vi "Final.vi"() -> ()   [LabVIEW 2017]
doc: "This example demonstrates how to read the hand position and velocity using the Leap Motion Controller."
uses:
  <vilib>/MakerHub/Leap/Private/Type Defs/Frame.ctl
  <vilib>/MakerHub/Leap/Private/Type Defs/Gesture Key Tap.ctl
  <vilib>/MakerHub/Leap/Private/Type Defs/Gesture Common.ctl
  <vilib>/MakerHub/Leap/Private/Type Defs/Gesture Type.ctl
  <vilib>/MakerHub/Leap/Private/Type Defs/Gesture State.ctl
  <vilib>/MakerHub/Leap/Private/Type Defs/Vector.ctl
  <vilib>/MakerHub/Leap/Private/Type Defs/Gesture Circle.ctl
  <vilib>/MakerHub/Leap/Private/Type Defs/Gesture Screen Tap.ctl
  <vilib>/MakerHub/Leap/Private/Type Defs/Gesture Swipe.ctl
  <vilib>/MakerHub/Leap/Private/Type Defs/Hand.ctl
  <vilib>/MakerHub/Leap/Private/Type Defs/Pointable.ctl
  <vilib>/MakerHub/Leap/Private/Type Defs/Pointable Type.ctl
  <vilib>/MakerHub/Leap/Private/Type Defs/Pointable Zone.ctl
  <vilib>/Instr/_visa.llb/VISA Configure Serial Port (Instr).vi
  <vilib>/MakerHub/Leap/Public/Instance VIs/Read 1 Hand Position Velocity.vi
  <vilib>/MakerHub/Leap/LMH-Leap.lvlib
panel:
  out "Hand XZ Position":cluster{"X":sgl, "Z":sgl, "Y":sgl}[](graph)
  out "Y Velocity (m/s) 2":sgl(slide) scale=2.0..-2.0
  out "X Velocity (m/s)":sgl(slide) scale=-2.0..2.0
  out "Z Velocity (m/s)":sgl(slide) scale=2.0..-2.0
  out "Hand XYZ Position":cluster{"X":sgl, "Y":sgl, "Z":sgl}
  out "error out":errorcluster
  out "error?":bool
  out "STRING_SEND_FINAL":string
  in  "COM Port":refnum<visa-resource-name>
  in  "baud rate (9600)":u32=9600
  in  "string":string
  out "Frame":T1
  out "Leap Connected?":bool
  in  "Stop Button":bool
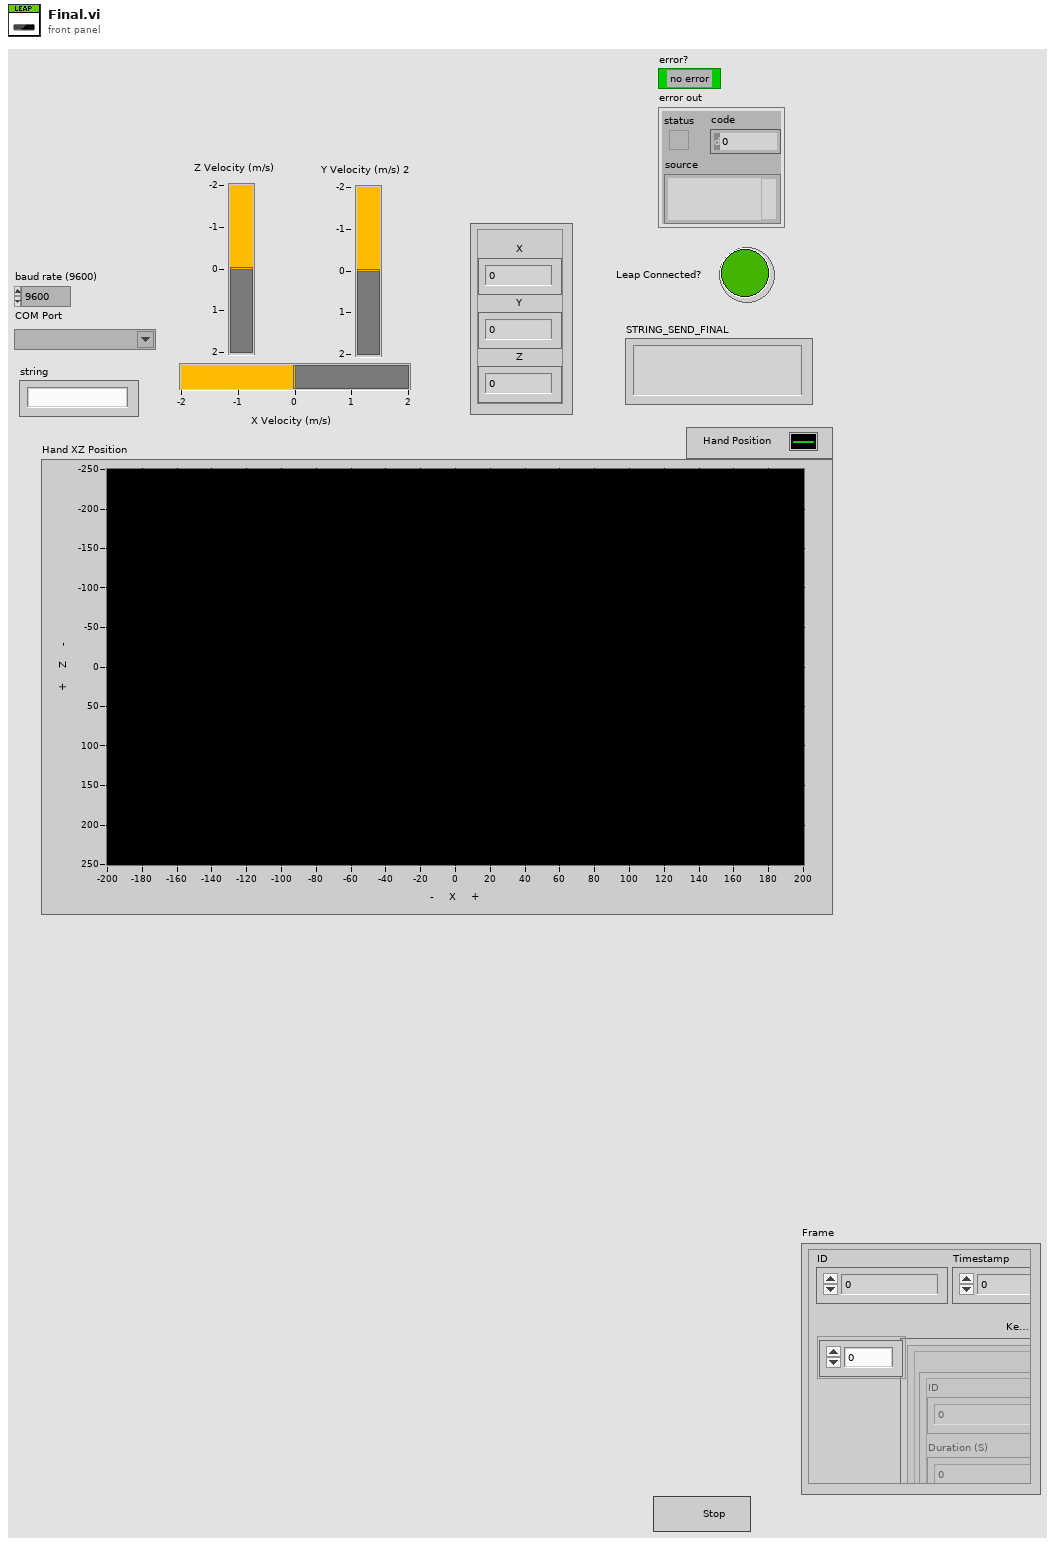
[diagram p1: front panel]
types:
  T1 = typedef "LMH-Leap.lvlib/Frame.ctl" = cluster{"ID":i64, "Timestamp":i64, "Current FPS":dbl, "Key Tap Gestures":T2[], "Circle Gestures":T7[], "Screen Tap Gestures":T8[], "Swipe Gestures":T9[], "Hands":T10[]}
  T2 = typedef "LMH-Leap.lvlib/Gesture Key Tap.ctl" = cluster{"Common":T3, "Direction":T6, "Position":T6, "Progress":dbl}
  T3 = typedef "LMH-Leap.lvlib/Gesture Common.ctl" = cluster{"ID":dbl, "Duration (S)":dbl, "Gesture Type":T4, "Gesture State":T5}
  T4 = typedef "LMH-Leap.lvlib/Gesture Type.ctl" = enum16{"Invalid", "Swipe", "Circle", "Screen Tap", "Key Tap"}
  T5 = typedef "LMH-Leap.lvlib/Gesture State.ctl" = enum16{"Invalid", "Start", "Update", "Stop"}
  T6 = typedef "LMH-Leap.lvlib/Vector.ctl" = cluster{"Pitch":sgl, "Yaw":sgl, "Roll":sgl, "Magnitude":sgl, "XYZ":sgl[]}
  T7 = typedef "LMH-Leap.lvlib/Gesture Circle.ctl" = cluster{"Common":T3, "Center":T6, "Normal":T6, "Progress":dbl, "Radius":dbl}
  T8 = typedef "LMH-Leap.lvlib/Gesture Screen Tap.ctl" = cluster{"Common":T3, "Direction":T6, "Position":T6, "Progress":dbl}
  T9 = typedef "LMH-Leap.lvlib/Gesture Swipe.ctl" = cluster{"Common":T3, "Direction":T6, "Position":T6, "Start Position":T6, "Speed":dbl}
  T10 = typedef "LMH-Leap.lvlib/Hand.ctl" = cluster{"Palm Normal":T6, "Palm Position":T6, "Palm Velocity":T6, "Direction":T6, "Palm Position (Stabilized)":T6, "Sphere Center":T6, "Pointables":T11[], "ID":i32, "Time Visible":sgl, "Sphere Radius":sgl}
  T11 = typedef "LMH-Leap.lvlib/Pointable.ctl" = cluster{"Type":T12, "Touch Zone":T13, "ID":i32, "Length":dbl, "Width":dbl, "Time Visible":dbl, "Touch Distance":dbl, "Direction":T6, "Tip Position":T6, "Tip Velocity":T6, "Tip Position (Stabilized)":T6}
  T12 = typedef "LMH-Leap.lvlib/Pointable Type.ctl" = enum16{"Finger", "Tool"}
  T13 = typedef "LMH-Leap.lvlib/Pointable Zone.ctl" = enum16{"None", "Hovering", "Touching"}
  T14 = typedef "LMH-Leap.lvlib/Leap Handle.ctl" = cluster{"LeapCSharp":refnum<k24>}
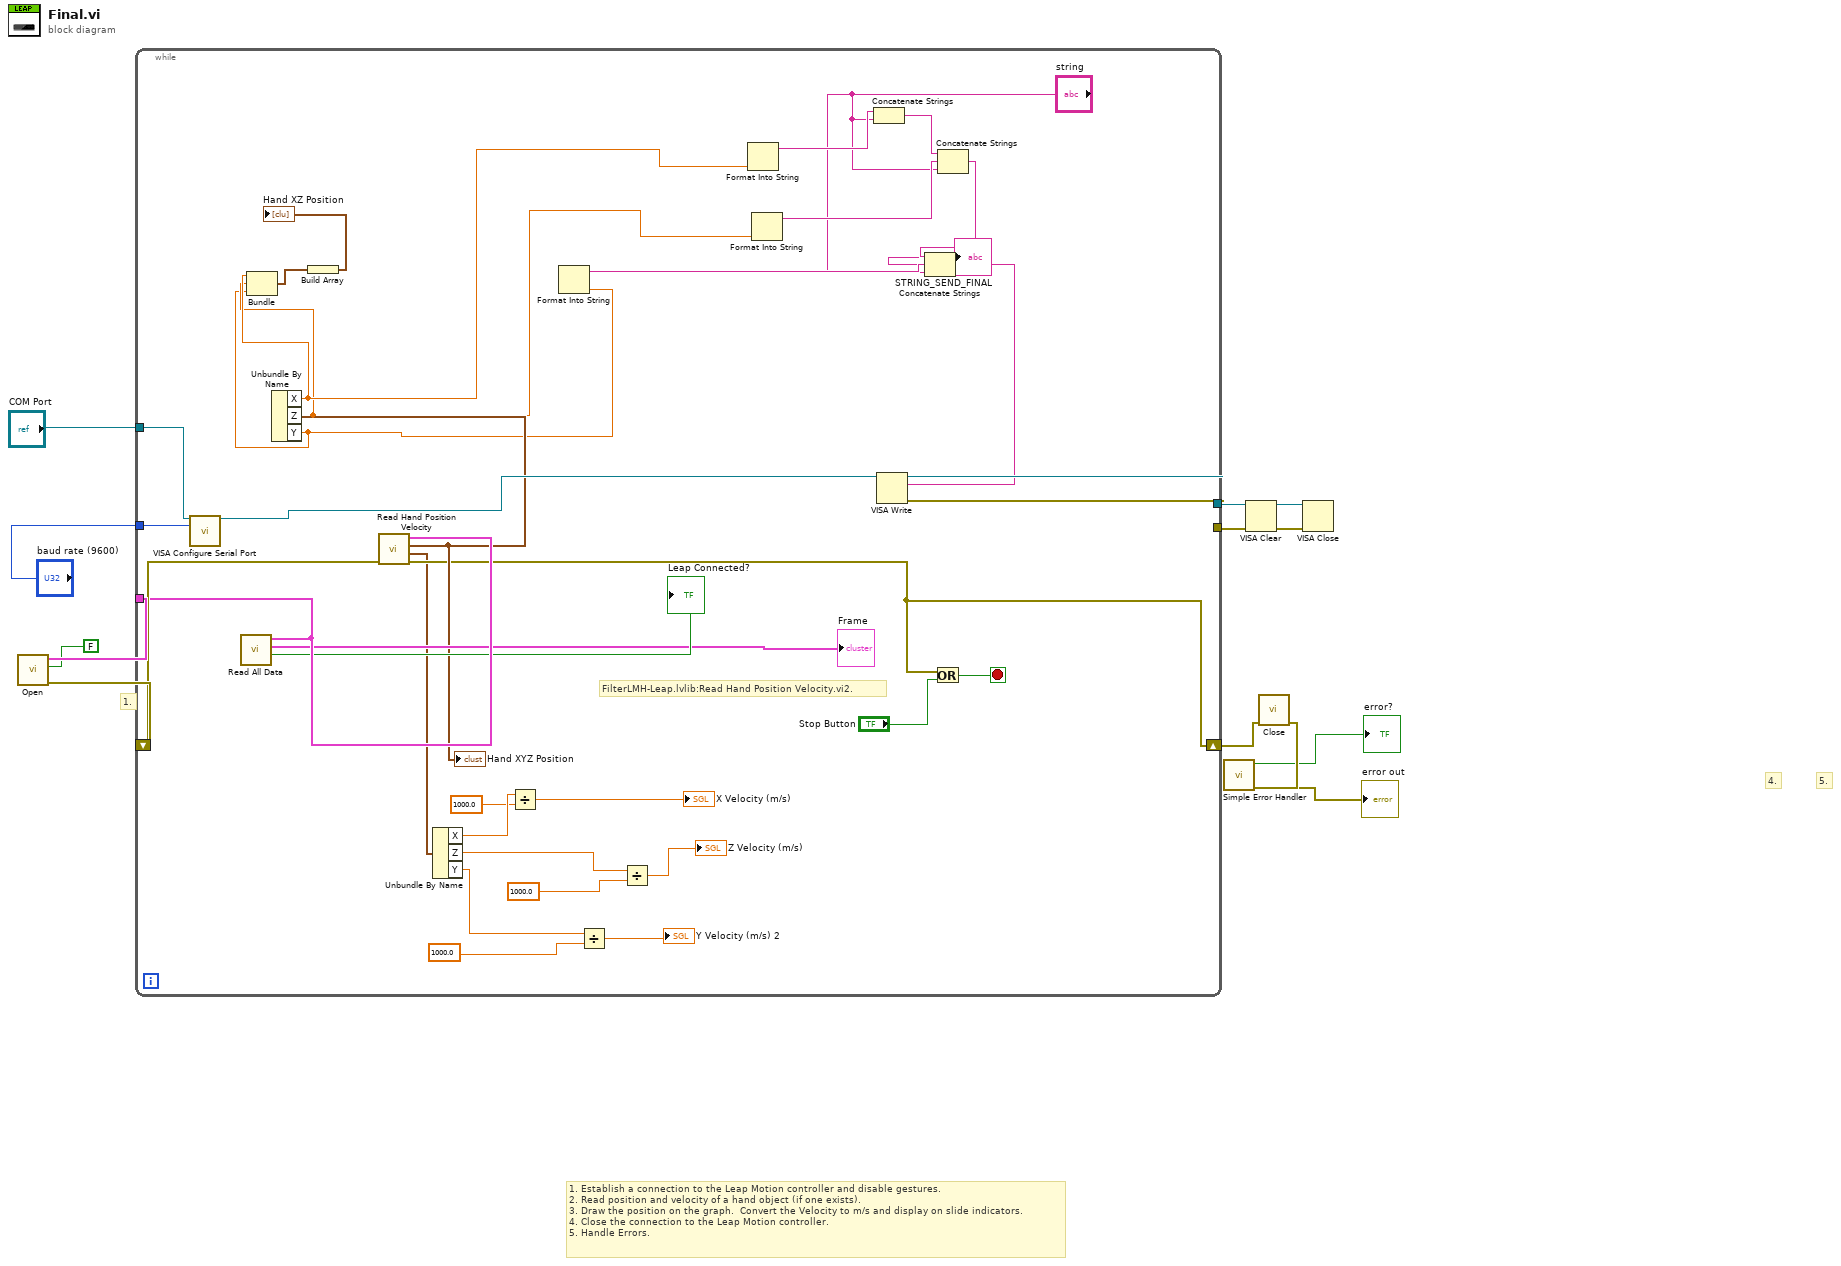
[diagram p0: block diagram]
diagram:
  # "1. Establish a connection to the Leap Motion controller and disable gestures.\n2. Read position and velocity of a hand object (if one exists).\n3. Draw the position on the graph.  Convert the Velocity to m/s and display on slide indicators.\n4. Close the connection to the Leap Motion controller.\n5. Handle Errors."
  # "5."
  # "4."
  # "1."
  n1 = call <vilib>:"Open.vi"("Enable Gestures? (T)"=FALSE) -> ("Error Out"=w12:errorcluster, "Leap Handle"=w13:T14)  [unwired: 9 in]
  n2 = while {
    tunnel: w13 -> [w45]
    shift-right: [w29] -> w4
    shift-left: w12 -> [w46]
    tunnel: [w42] -> w8
    tunnel: [w41] -> w6
    tunnel: "COM Port" -> [w40]
    tunnel: "baud rate (9600)" -> [w39]
    stop <- w48 stop-if-true
    # "FilterLMH-Leap.lvlib:Read Hand Position Velocity.vi2."
    n3 = call-poly "VISA Configure Serial Port"("VISA resource name"=w40, "baud rate (9600)"=w39) -> ("VISA resource name out"=w38:refnum<visa-resource-name>)  [unwired: 12 in, 1 out]
    n4 = call <vilib>:"Read All Data.vi"("Leap Handle"=w45) -> ("Leap Connected?"=→"Leap Connected?":bool, "Frame"=→"Frame":T1)  [unwired: 7 in, 2 out]
    n5 = call-poly <vilib>:"Read Hand Position Velocity.vi"("Error In"=w46, "Leap Handle"=w45) -> ("Error Out"=w29:errorcluster, "Hand Velocity"=w22:cluster{"X":sgl, "Y":sgl, "Z":sgl}, "Hand Position"=w30:cluster{"X":sgl, "Y":sgl, "Z":sgl})  [unwired: 6 in, 1 out]
    "Hand XYZ Position" <- w30
    n6 = Unbundle By Name(w30) -> ("X"=w18:sgl, "Z"=w17:sgl, "Y"=w16:sgl)
    n7 = Bundle("X"=w18, "Z"=w17, "Y"=w16) -> (w15:cluster{"X":sgl, "Z":sgl, "Y":sgl})  [unwired: 1 in]
    n8 = Build Array(w15) -> (→"Hand XZ Position":cluster{"X":sgl, "Z":sgl, "Y":sgl}[])
    n9 = Unbundle By Name(w22) -> ("X"=w26:sgl, "Z"=w28:sgl, "Y"=w21:sgl)
    n10 = Divide(x=w26, y=sgl 1000.0) -> (x/y=→"X Velocity (m/s)":sgl)
    n11 = Format Into String(w16) -> (resulting string=w33:string)  [unwired: 3 in, 1 out]
    n12 = Divide(x=w21, y=sgl 1000.0) -> (x/y=→"Y Velocity (m/s) 2":sgl)
    n13 = Divide(x=w28, y=sgl 1000.0) -> (x/y=→"Z Velocity (m/s)":sgl)
    n14 = Format Into String(w18) -> (resulting string=w37:string)  [unwired: 3 in, 1 out]
    n15 = Format Into String(w17) -> (resulting string=w35:string)  [unwired: 3 in, 1 out]
    n16 = Concatenate Strings(w37, "string") -> (w36:string)
    n17 = Or(x=w29, y="Stop Button") -> (x .or. y?=w48:bool)
    n18 = Concatenate Strings(w36, w35, "string") -> (w34:string)
    n19 = Concatenate Strings(w34, w33, "string") -> (w31:string)
    "STRING_SEND_FINAL" <- w31
    n20 = VISA Write(VISA resource name=w38, write buffer=w31) -> (VISA resource name out=w42:refnum<visa-resource-name>, error out=w41:errorcluster)  [unwired: 1 in, 1 out]
  }
  n21 = VISA Clear(VISA resource name=w8, error in (no error)=w6) -> (VISA resource name out=w7:refnum<visa-resource-name>, error out=w5:errorcluster)
  n22 = call <vilib>:"Close.vi"("Error In"=w4) -> ("Error Out"=w3:errorcluster)  [unwired: 10 in]
  n23 = call <vilib>:"Simple Error Handler.vi"("error in (no error)"=w3) -> ("error?"=→"error?":bool, "error out"=→"error out":errorcluster)  [unwired: 4 in, 3 out]
  n24 = VISA Close(VISA resource name=w7, error in (no error)=w5) -> ()  [unwired: 1 out]
